vi "ParseArguments.vi"(8 "error in (no error)":errorcluster, 10 "Inputs":string[](array[string]), 11 "ExecuteMultipleBuildSpecs in":refnum<class "ExecuteMultipleBuildSpecs.lvclass">) -> (0 "error out":errorcluster, 3 "ExecuteMultipleBuildSpecs out":refnum<class "ExecuteMultipleBuildSpecs.lvclass">)   [LabVIEW 2014, in "ExecuteMultipleBuildSpecs.lvclass"]
uses:
  ExecuteMultipleBuildSpecs.lvclass
  ExecuteMultipleBuildSpecs.lvclass/ExecuteMultipleBuildSpecs.ctl
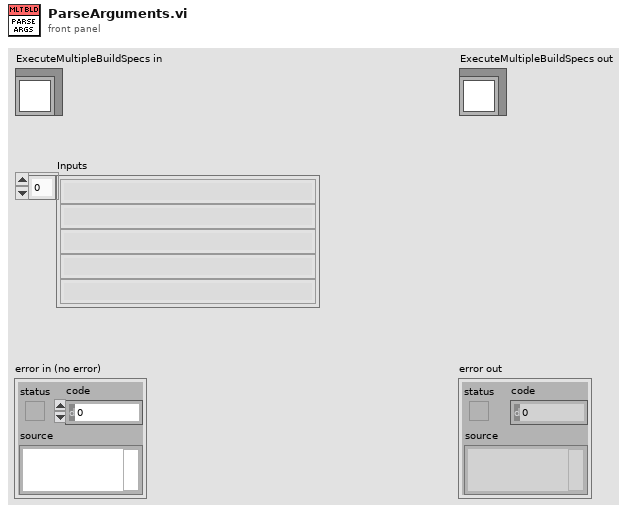
[diagram p1: front panel]
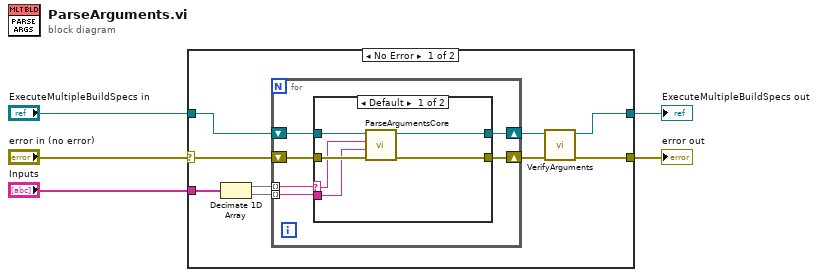
[diagram p0: block diagram]
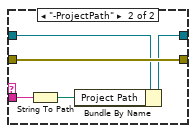
[diagram p2: hidden frame]
diagram:
  n1 = case shown="No Error" "error in (no error)" {
    selector: "error in (no error)" -> [w12 w33]
    tunnel: [w14 w33] -> w4
    tunnel: [w13 w32] -> w2
    tunnel: "ExecuteMultipleBuildSpecs in" -> [w10 w32]
    tunnel: "Inputs" -> [w8 _]
    frame No Error {
      n2 = Decimate 1D Array(w8) -> (w7:string[], w6:string[])
      n3 = for {
        shift-right: [w19] -> w11
        shift-left: w12 -> [w20]
        shift-right: [w17] -> w9
        shift-left: w10 -> [w18]
        tunnel: w7 -> [w16] mode=indexing
        tunnel: w6 -> [w15] mode=indexing
        n4 = case shown="Default" w16 {
          selector: w16 -> [w22 _]
          tunnel: w20 -> [w26 w31]
          tunnel: [w25 w31] -> w19
          tunnel: w15 -> [w21 w30]
          tunnel: w18 -> [w24 w28]
          tunnel: [w23 w27] -> w17
          frame Default {
            n5 = call-dynamic "ParseArgumentsCore.vi"("error in (no error)"=w26, "Value"=w21, "Option"=w22, "ExecuteMultipleBuildSpecs in"=w24) -> ("error out"=w25:errorcluster, "ExecuteMultipleBuildSpecs out"=w23:refnum<class "ExecuteMultipleBuildSpecs.lvclass">)  [unwired: 6 in]
          }
          frame "-ProjectPath" {
            n6 = String To Path(string=w30) -> (path=w29:path)
            n7 = Bundle By Name(cluster=w28, "Project Path"=w29) -> (w27:refnum<class "ExecuteMultipleBuildSpecs.lvclass">)
          }
        }
      }
      n8 = call "VerifyArguments.vi"("error in (no error)"=w11, "ExecuteMultipleBuildSpecs in"=w9) -> ("error out"=w14:errorcluster, "ExecuteMultipleBuildSpecs out"=w13:refnum<class "ExecuteMultipleBuildSpecs.lvclass">)  [unwired: 8 in]
    }
    frame Error {
    }
  }
  "error out" <- w4
  "ExecuteMultipleBuildSpecs out" <- w2
